vi "лаба 2.vi"() -> ()   [LabVIEW 2013]
panel:
  in  "Input 4":T1
  in  "Input 3":T1
  in  "Input 2":T1
  in  "Input 1":T1
  in  "Input 0":T1
  out "Output 4":T2
  out "Output 3":T2
  out "Output 2":T2
  out "Output 1":T2
  out "Output 0":T2
  out "Output":T2
  in  "Input":T1
  in  "Adress":T3
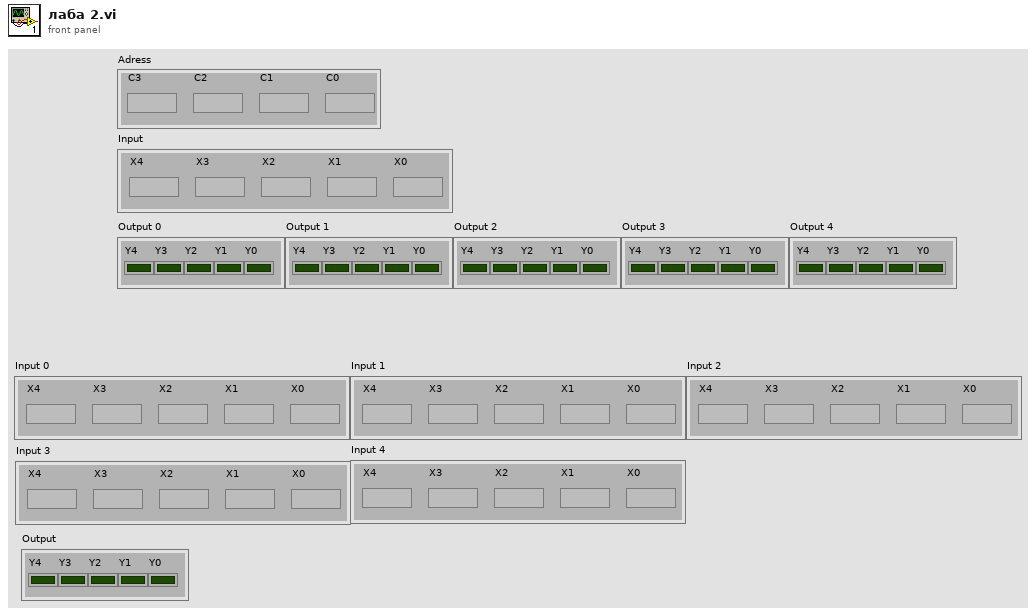
[diagram p1: front panel]
types:
  T1 = cluster{"X1":bool, "X4":bool, "X3":bool, "X2":bool, "X0":bool}
  T2 = cluster{"Y4":bool, "Y3":bool, "Y2":bool, "Y1":bool, "Y0":bool}
  T3 = cluster{"С3":bool, "С2":bool, "С1":bool, "С0":bool}
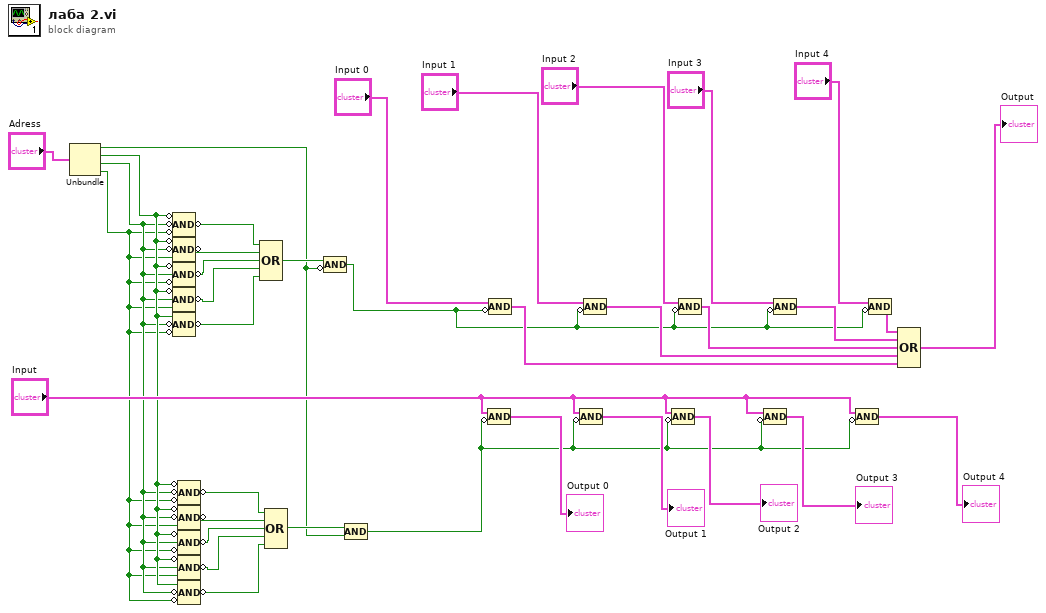
[diagram p0: block diagram]
diagram:
  n1 = Unbundle("Adress") -> ("С3"=w3:bool, "С2"=w6:bool, "С1"=w5:bool, "С0"=w4:bool)
  n2 = Compound Arithmetic op=AND(invert w6, invert w5, invert w4) -> (invert w18:bool)
  n3 = Compound Arithmetic op=AND(invert w6, invert w5, w4) -> (invert w17:bool)
  n4 = Compound Arithmetic op=AND(invert w6, w5, invert w4) -> (invert w16:bool)
  n5 = Compound Arithmetic op=AND(invert w6, w5, w4) -> (invert w15:bool)
  n6 = Compound Arithmetic op=AND(w6, invert w5, invert w4) -> (invert w14:bool)
  n7 = Compound Arithmetic op=AND(invert w6, invert w5, invert w4) -> (invert w13:bool)
  n8 = Compound Arithmetic op=AND(invert w6, invert w5, w4) -> (invert w12:bool)
  n9 = Compound Arithmetic op=AND(invert w6, w5, invert w4) -> (invert w11:bool)
  n10 = Compound Arithmetic op=AND(invert w6, w5, w4) -> (invert w10:bool)
  n11 = Compound Arithmetic op=AND(w6, invert w5, invert w4) -> (invert w9:bool)
  n12 = Compound Arithmetic op=OR(w18, w17, w16, w15, w14) -> (w7:bool)
  n13 = Compound Arithmetic op=OR(w13, w12, w11, w10, w9) -> (w8:bool)
  n14 = Compound Arithmetic op=AND(w7, invert w3) -> (w2:bool)
  n15 = Compound Arithmetic op=AND(w8, w3) -> (w1:bool)
  n16 = Compound Arithmetic op=AND("Input", invert w1) -> (→"Output 0":T1)
  n17 = Compound Arithmetic op=AND("Input 0", invert w2) -> (w26:T1)
  n18 = Compound Arithmetic op=AND("Input", invert w1) -> (→"Output 1":T1)
  n19 = Compound Arithmetic op=AND("Input 1", invert w2) -> (w27:T1)
  n20 = Compound Arithmetic op=AND("Input", invert w1) -> (→"Output 2":T1)
  n21 = Compound Arithmetic op=AND("Input 2", invert w2) -> (w28:T1)
  n22 = Compound Arithmetic op=AND("Input", invert w1) -> (→"Output 3":T1)
  n23 = Compound Arithmetic op=AND("Input 3", invert w2) -> (w29:T1)
  n24 = Compound Arithmetic op=AND("Input", invert w1) -> (→"Output 4":T1)
  n25 = Compound Arithmetic op=AND("Input 4", invert w2) -> (w30:T1)
  n26 = Compound Arithmetic op=OR(w30, w29, w28, w27, w26) -> (→"Output":T1)
